vi "31_part_of_image.vi"() -> ()   [LabVIEW 2018]
uses:
  <vilib>/vision/NI_Vision_Development_Module.lvlib
panel:
  out "Numeric":u8
  out "Image Pixels (U8) 2":u8[](array[numeric])
  out "Image 2":T1(plugin-control)
  out "Image Pixels (U8)":u8[][](array[numeric])
  in  "stop":bool
  out "Image":T1(plugin-control)
  # "提取選取部份"
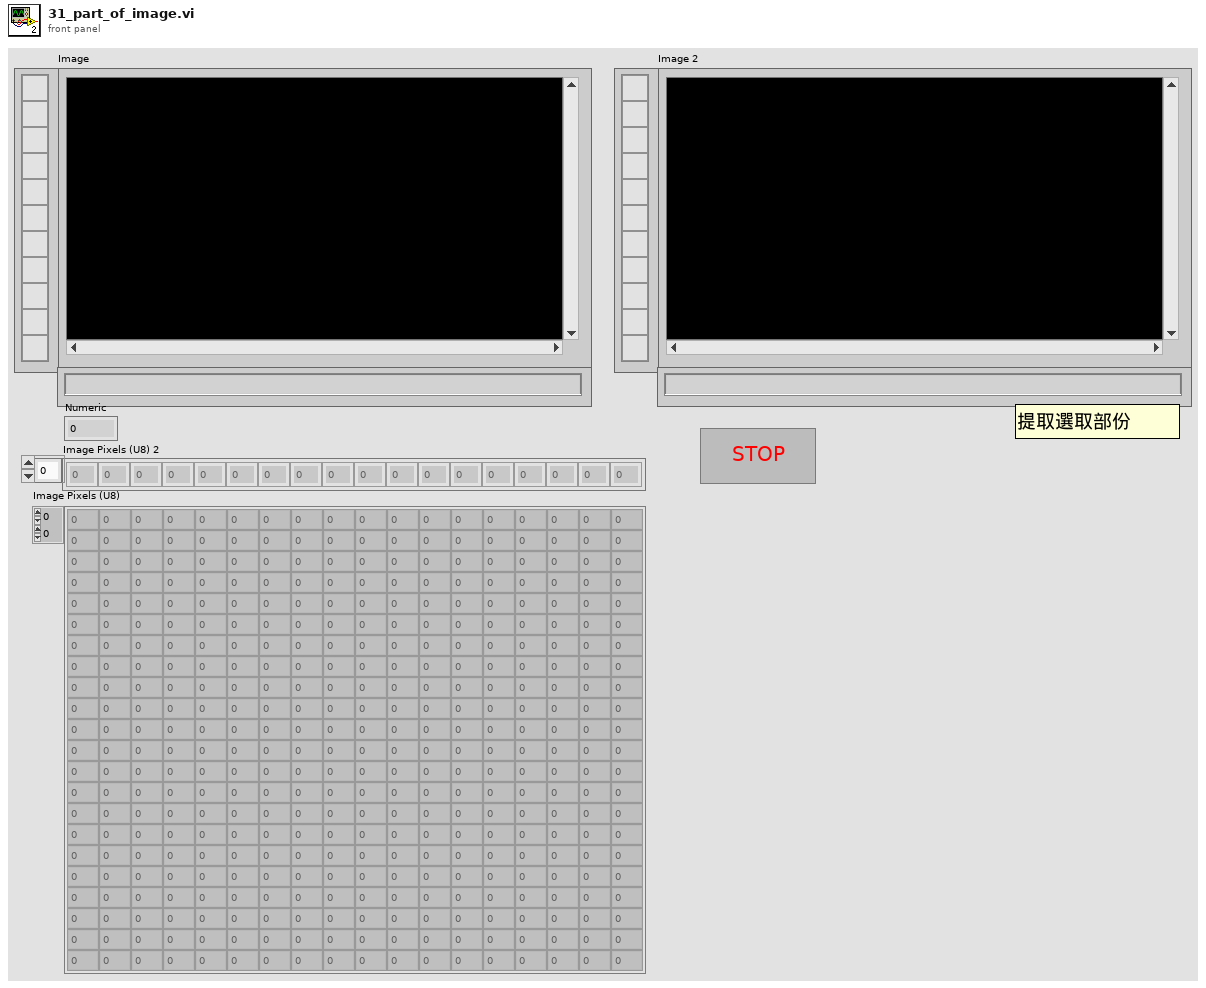
[diagram p1: front panel]
types:
  T1 = typedef "IMAQ Image.ctl" = refnum<image>
  T2 = typedef "Image Type" = u32
  T3 = cluster{"Global Rectangle":i32[], "Contours":cluster{"Contour Type":u32, "ROI Type":u32, "Points":i32[]}[]}
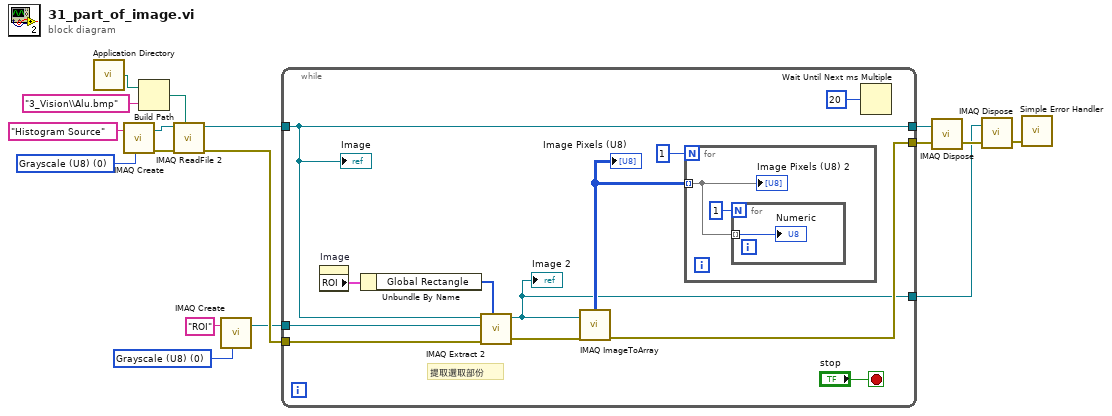
[diagram p0: block diagram]
diagram:
  w7 = T2 0 items=["Grayscale (U8)", "Grayscale (I16)", "Grayscale (SGL)", "Complex (CSG)", "RGB (U32)", "HSL (U32)", "RGB (U64)", "Grayscale (U16)"] ("Image Type")
  w8 = T2 0 items=["Grayscale (U8)", "Grayscale (I16)", "Grayscale (SGL)", "Complex (CSG)", "RGB (U32)", "HSL (U32)", "RGB (U64)", "Grayscale (U16)"] ("Image Type")
  n1 = call <vilib>:"Application Directory.vi"() -> ("Application Directory"=w10:path)
  n2 = call "IMAQ Create"("Image Name"="Histogram Source", "Image Type"=w8) -> ("New Image"=w17:T1, "error out"=w16:errorcluster)  [unwired: 3 in]
  n3 = Build Path(base path=w10, name or relative path="3_Vision\\Alu.bmp") -> (appended path=w11:path)
  n4 = call "IMAQ ReadFile 2"("File Path"=w11, "error in (no error)"=w16, "Image"=w17) -> ("error out"=w12:errorcluster, "Image Out"=w14:T1)  [unwired: 4 in, 3 out]
  n5 = call "IMAQ Create"("Image Name"="ROI", "Image Type"=w7) -> ("New Image"=w5:T1)  [unwired: 3 in, 1 out]
  n6 = while {
    tunnel: w14 -> [w25]
    tunnel: [w25] -> w13
    tunnel: w12 -> [w22]
    tunnel: w5 -> [w24]
    tunnel: [w27] -> w4
    tunnel: [w18] -> w1
    stop <- "stop" stop-if-true
    # "提取選取部份"
    n7 = property on="Image" class="ImageControl"() -> ("ROI"=w26:T3)  [unwired: 2 in, 2 out]
    n8 = Unbundle By Name "Unbundle By Name"(w26) -> ("Global Rectangle"=w23:i32[])
    n9 = call "IMAQ Extract 2"("Optional Rectangle"=w23, "error in (no error)"=w22, "Image Dst"=w24, "Image Src"=w25) -> ("error out"=w21:errorcluster, "Image Dst Out"=w18:T1)  [unwired: 6 in]
    "Image 2" <- w18
    n10 = call "IMAQ ImageToArray"("error in (no error)"=w21, "Image"=w18) -> ("error out"=w27:errorcluster, "Image Pixels (U8)"=w19:u8[][])  [unwired: 2 in, 3 out]
    "Image Pixels (U8)" <- w19
    n11 = for {
      N: 1 -> [_]
      tunnel: w19 -> [w30] mode=indexing
      n12 = for {
        N: 1 -> [_]
        tunnel: w30 -> [w32] mode=indexing
        "Numeric" <- w32
      }
      "Image Pixels (U8) 2" <- w30
    }
    n13 = Wait Until Next ms Multiple(millisecond multiple=u32 20) -> ()  [unwired: 1 out]
    "Image" <- w25
  }
  n14 = call "IMAQ Dispose"("Image"=w13, "error in (no error)"=w4) -> ("error out"=w3:errorcluster)  [unwired: 4 in]
  n15 = call "IMAQ Dispose"("Image"=w1, "error in (no error)"=w3) -> ("error out"=w2:errorcluster)  [unwired: 4 in]
  n16 = call <vilib>:"Simple Error Handler.vi"("error in (no error)"=w2) -> ()  [unwired: 4 in, 5 out]
